vi "S7-PPI协议.vi"() -> ()   [LabVIEW 2014]
uses:
  <vilib>/Instr/_visa.llb/VISA Configure Serial Port (Instr).vi
panel:
  out "RVW34":u16
  out "RVW32":u16
  out "RVW30":u16
  out "RVW28":u16
  out "RVW26":u16
  out "RVW24":u16
  out "RVW22":u16
  out "RVW20":u16
  out "RVW18":u16
  out "RVW16":u16
  out "RVW14":u16
  out "RVW12":u16
  out "RVW10":u16
  out "RVW8":u16
  out "RVW6":u16
  out "RVW4":u16
  out "RVW2":u16
  out "RVW0":u16
  in  "VW34":u16
  in  "VW32":u16
  in  "VW30":u16
  in  "VW28":u16
  in  "VW26":u16
  in  "VW24":u16
  in  "VW22":u16
  in  "VW20":u16
  in  "VW18":u16
  in  "VW16":u16
  in  "VW14":u16
  in  "VW12":u16
  in  "VW10":u16
  in  "VW8":u16
  in  "VW6":u16
  in  "VW4":u16
  in  "VW2":u16
  in  "VW0":u16
  out "值 3":u32
  out "Q3.0":bool
  out "Q3.1":bool
  out "Q3.2":bool
  out "Q3.3":bool
  out "Q3.4":bool
  out "Q3.5":bool
  out "Q3.6":bool
  out "Q3.7":bool
  out "M2.0":bool
  out "M2.1":bool
  out "M2.2":bool
  out "M2.4":bool
  out "M2.3":bool
  out "M2.5":bool
  out "M2.6":bool
  out "M2.7":bool
  out "M1.0":bool
  out "M1.1":bool
  out "M1.2":bool
  out "M1.3":bool
  out "M1.4":bool
  out "M1.5":bool
  out "M1.6":bool
  out "M1.7":bool
  out "M0.0":bool
  out "M0.1":bool
  out "M0.2":bool
  out "M0.3":bool
  out "M0.4":bool
  out "M0.5":bool
  out "M0.6":bool
  out "M0.7":bool
  in  "Q3.0":bool
  in  "Q3.1":bool
  in  "Q3.2":bool
  in  "Q3.3":bool
  in  "Q3.4":bool
  in  "Q3.5":bool
  in  "Q3.6":bool
  in  "Q3.7":bool
  in  "M2.0":bool
  in  "M2.1":bool
  in  "M2.2":bool
  in  "M2.3":bool
  in  "M2.4":bool
  in  "M2.5":bool
  in  "M2.6":bool
  in  "M2.7":bool
  in  "M1.0":bool
  in  "M1.1":bool
  in  "M1.2":bool
  in  "M1.3":bool
  in  "M1.4":bool
  in  "M1.5":bool
  in  "M1.6":bool
  in  "M1.7":bool
  in  "M0.0":bool
  in  "M0.1":bool
  in  "M0.2":bool
  in  "M0.3":bool
  in  "M0.4":bool
  in  "M0.5":bool
  in  "M0.6":bool
  in  "M0.7":bool
  out "值 2":u32
  in  "Q3.0":bool
  in  "Q3.1":bool
  in  "Q3.2":bool
  in  "Q3.3":bool
  in  "Q3.4":bool
  in  "Q3.5":bool
  in  "Q3.6":bool
  in  "Q3.7":bool
  in  "Q2.0":bool
  in  "Q2.1":bool
  in  "Q2.2":bool
  in  "Q2.3":bool
  in  "Q2.4":bool
  in  "Q2.5":bool
  in  "Q2.6":bool
  in  "Q2.7":bool
  in  "Q1.7":bool
  in  "Q1.6":bool
  in  "Q1.5":bool
  in  "Q1.4":bool
  in  "Q1.3":bool
  in  "Q1.2":bool
  in  "Q1.1":bool
  in  "Q1.0":bool
  in  "Q0.7":bool
  in  "Q0.6":bool
  in  "Q0.5":bool
  in  "Q0.4":bool
  in  "Q0.3":bool
  in  "Q0.2":bool
  in  "Q0.1":bool
  in  "Q0.0":bool
  out "Q3.0":bool
  out "Q3.1":bool
  out "Q3.2":bool
  out "Q3.3":bool
  out "Q3.4":bool
  out "Q3.5":bool
  out "Q3.6":bool
  out "Q3.7":bool
  out "Q2.0":bool
  out "Q2.1":bool
  out "Q2.2":bool
  out "Q2.4":bool
  out "Q2.3":bool
  out "Q2.5":bool
  out "Q2.6":bool
  out "Q2.7":bool
  out "Q1.0":bool
  out "Q1.1":bool
  out "Q1.2":bool
  out "Q1.3":bool
  out "Q1.4":bool
  out "Q1.5":bool
  out "Q1.6":bool
  out "Q1.7":bool
  out "Q0.0":bool
  out "Q0.1":bool
  out "Q0.2":bool
  out "Q0.3":bool
  out "Q0.4":bool
  out "Q0.5":bool
  out "Q0.6":bool
  out "Q0.7":bool
  out "I3.0":bool
  out "I3.1":bool
  out "I3.2":bool
  out "I3.3":bool
  out "I3.4":bool
  out "I3.5":bool
  out "I3.6":bool
  out "I3.7":bool
  out "I2.0":bool
  out "I2.1":bool
  out "I2.2":bool
  out "I2.4":bool
  out "I2.3":bool
  out "I2.5":bool
  out "I2.6":bool
  out "I2.7":bool
  out "I1.0":bool
  out "I1.1":bool
  out "I1.2":bool
  out "I1.3":bool
  out "I1.4":bool
  out "I1.5":bool
  out "I1.6":bool
  out "I1.7":bool
  out "I0.0":bool
  out "I0.1":bool
  out "I0.2":bool
  out "I0.3":bool
  out "I0.4":bool
  out "I0.5":bool
  out "I0.6":bool
  out "I0.7":bool
  in  "枚举":T1
  in  "读写时间":u32
  in  "baud":u32=9600 caption="波特率"
  in  "COM":refnum<visa-resource-name> caption="端口"
  in  "停止":bool
  in  "STOP":bool
  in  "RUN":bool
  # "I0.0-I0.7"
  # "I1.0-I1.7"
  # "I2.0-I2.7"
  # "I3.0-I3.7"
  # "https://item.taobao.com/item.htm?id=520867234520"
  # "Q0.0-Q0.7"
  # "Q1.0-Q1.7"
  # "Q2.0-Q2.7"
  # "Q3.0-Q3.7"
  # "本程序密码：635410@ ，已经由楼上的工具破解"
  # "M0.0-M0.7"
  # "M1.0-M1.7"
  # "M2.0-M2.7"
  # "M3.0-M3.7"
  # "运行前请选择正确的通讯端口，和\n波特率。注意读写扫描时间的填写\n此程序PLC默认地址为2，其他不能\n通讯连接。"
  # "注意：1:波特率19.2请将读写时间设置大于80，波特率9600请将读写时间设置大于200，禁止187.5运行,建议19.2kbt/s"
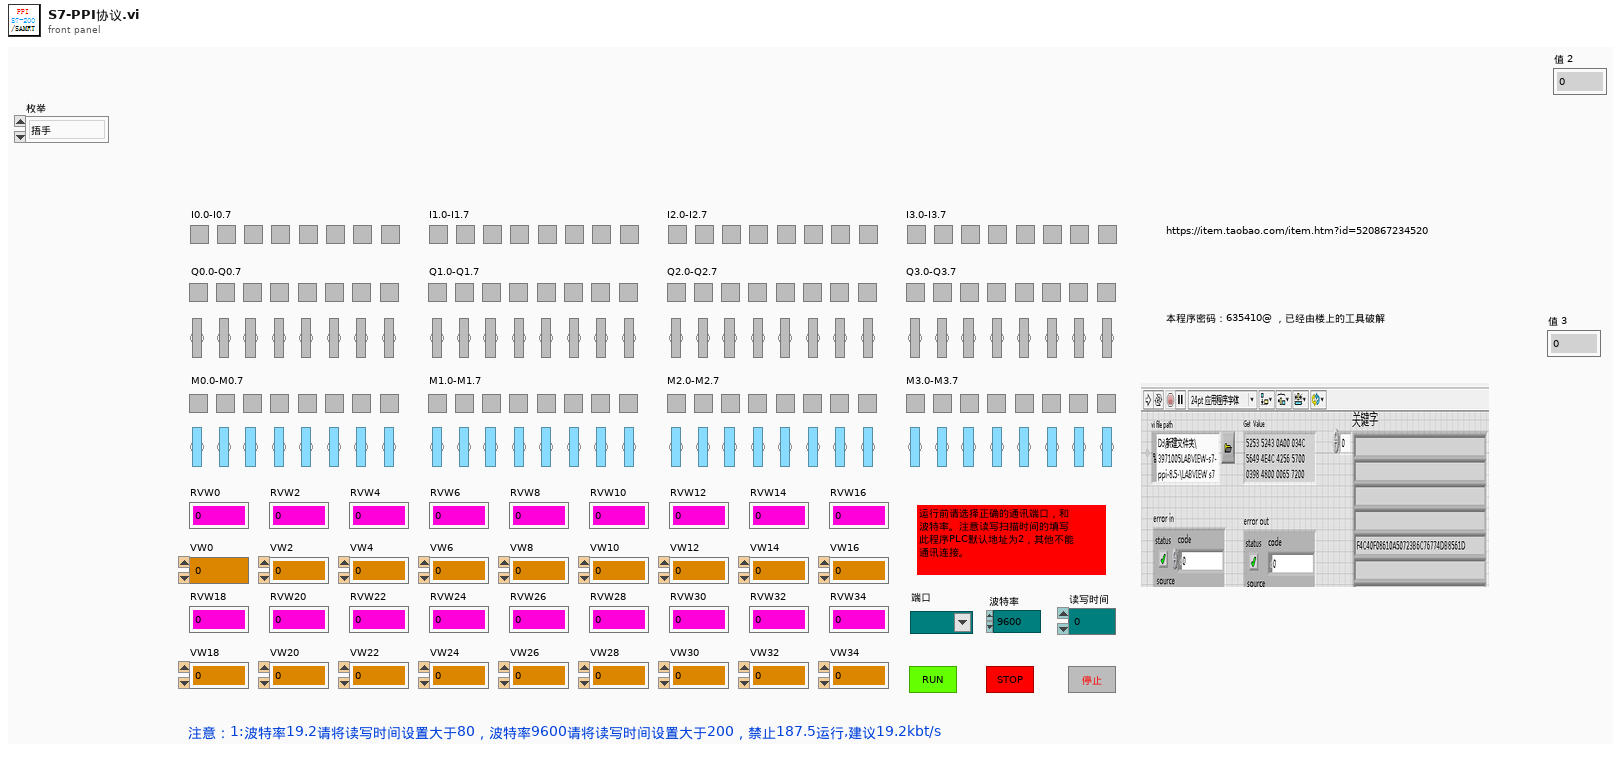
[diagram p1: front panel]
types:
  T1 = typedef "读取值枚举索引.ctl" = enum16{"捂手", "RUN", "STOP", "枚举RI", "枚举RQ", "枚举RM", "枚举RVW", "WID0", "WQD0", "WMD0", "WV"}
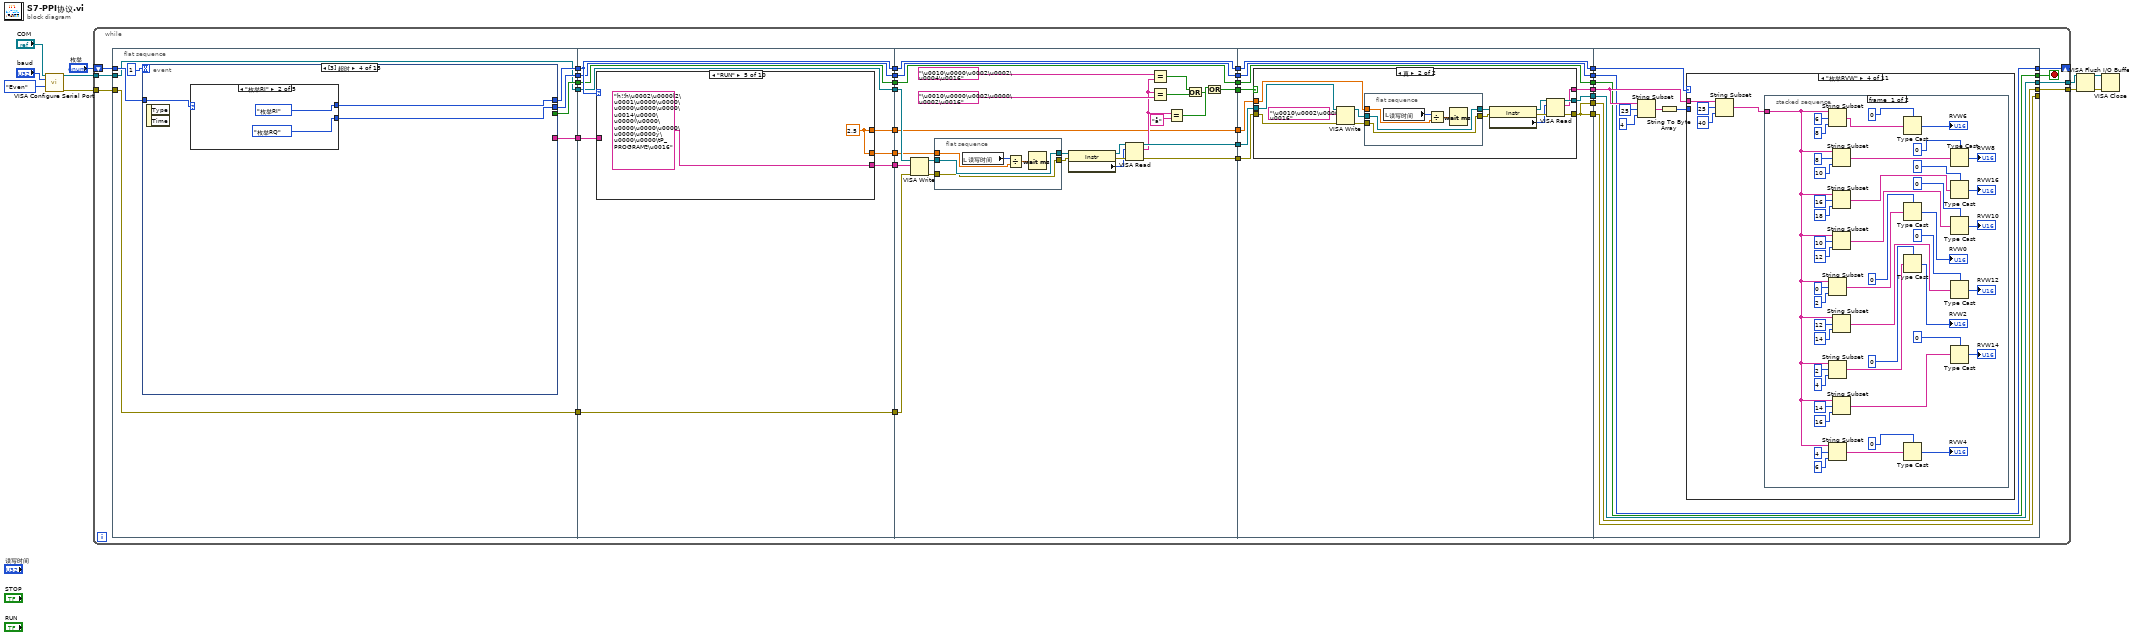
[diagram p0: block diagram]
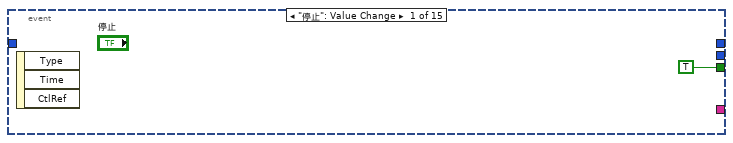
[diagram p2: hidden frame]
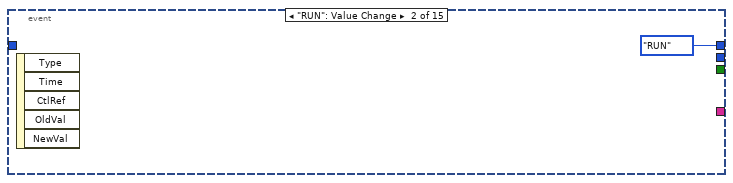
[diagram p3: hidden frame]
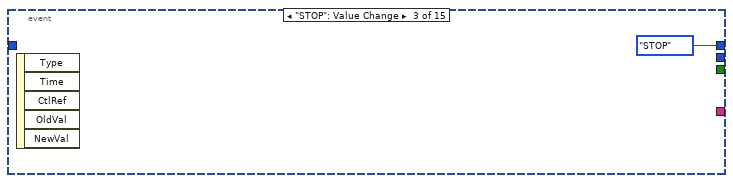
[diagram p4: hidden frame]
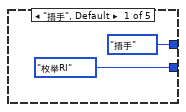
[diagram p5: hidden frame]
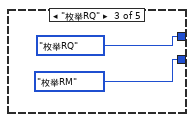
[diagram p6: hidden frame]
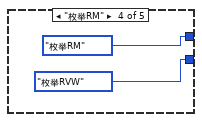
[diagram p7: hidden frame]
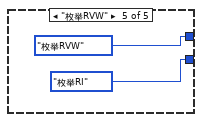
[diagram p8: hidden frame]
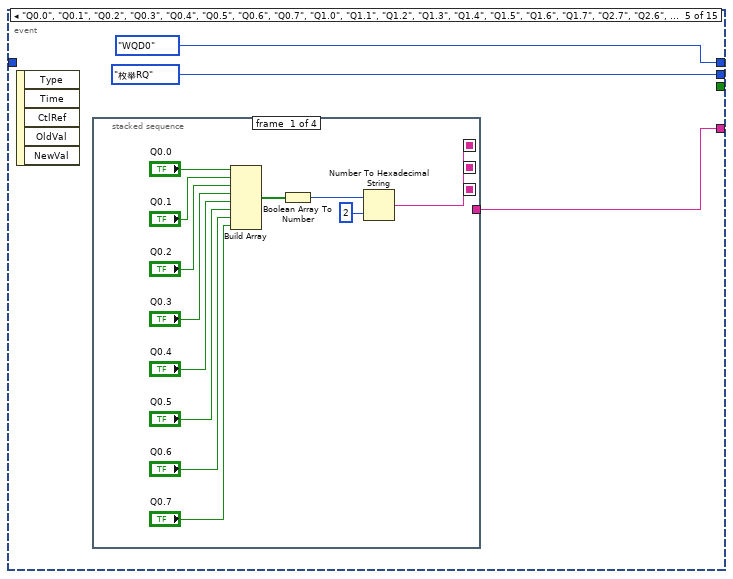
[diagram p9: hidden frame]
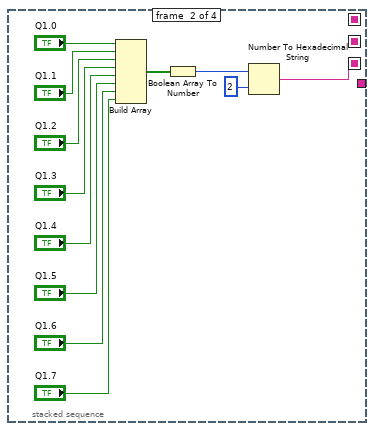
[diagram p10: hidden frame]
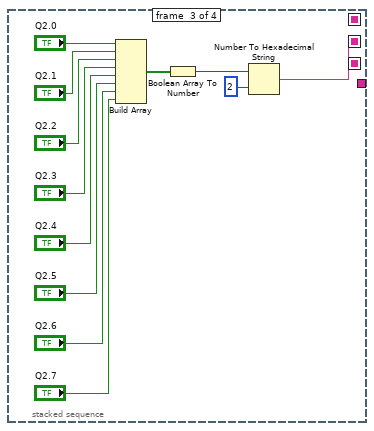
[diagram p11: hidden frame]
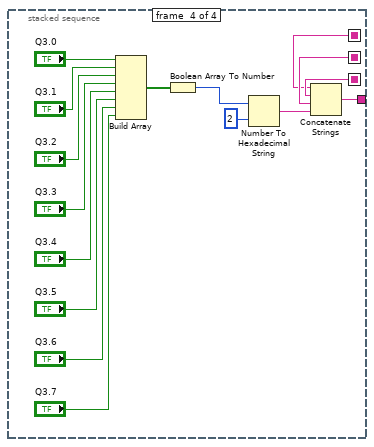
[diagram p12: hidden frame]
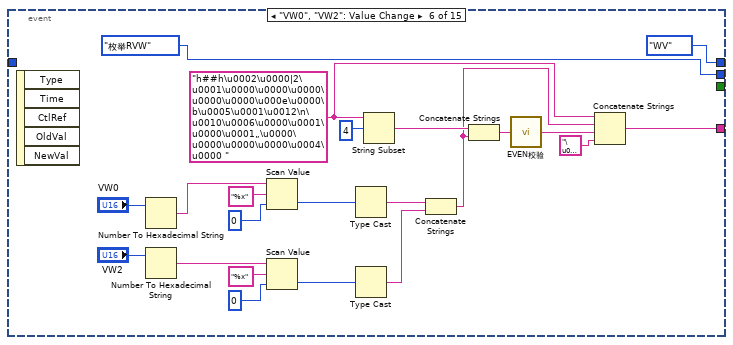
[diagram p13: hidden frame]
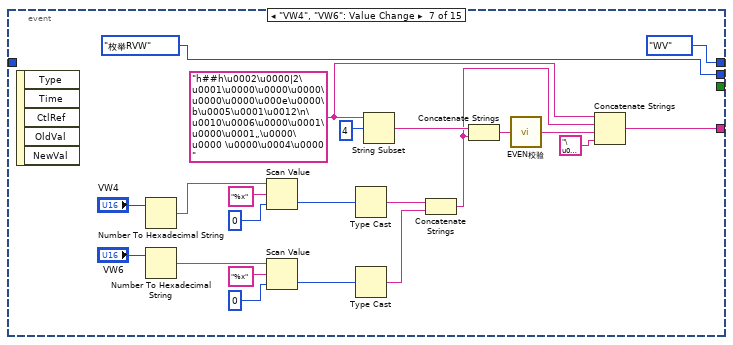
[diagram p14: hidden frame]
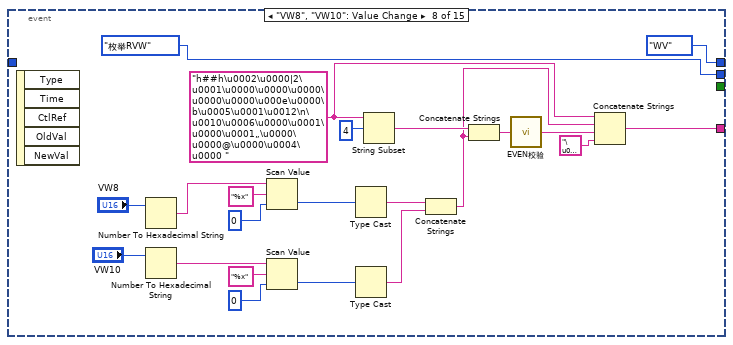
[diagram p15: hidden frame]
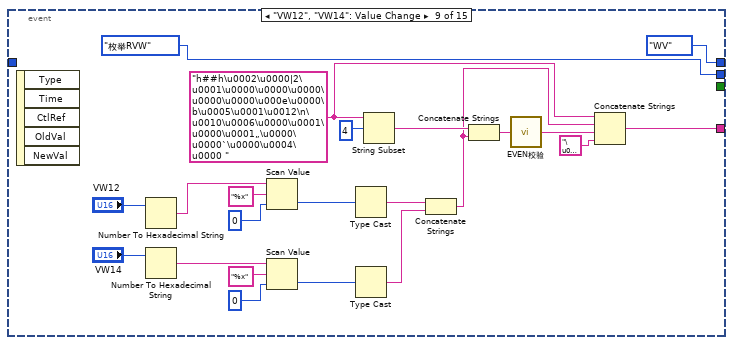
[diagram p16: hidden frame]
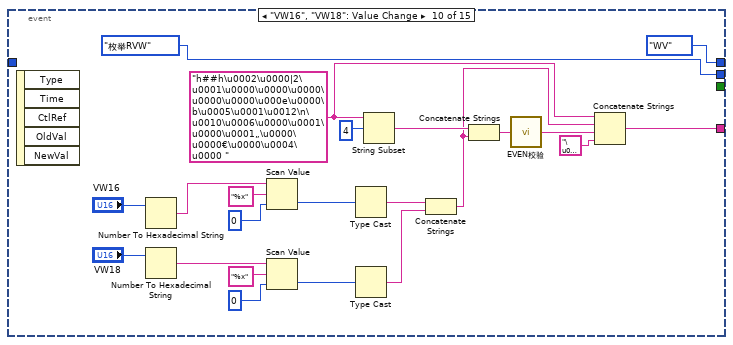
[diagram p17: hidden frame]
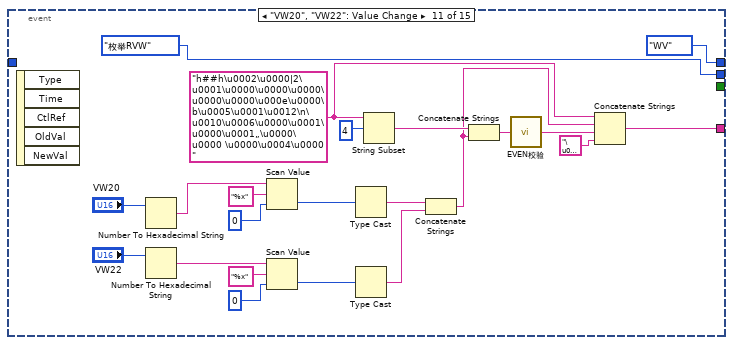
[diagram p18: hidden frame]
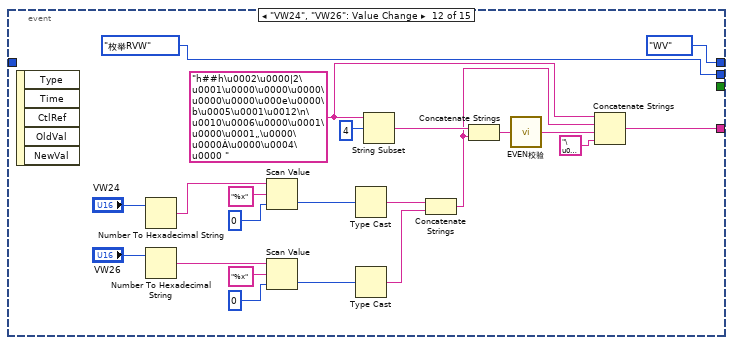
[diagram p19: hidden frame]
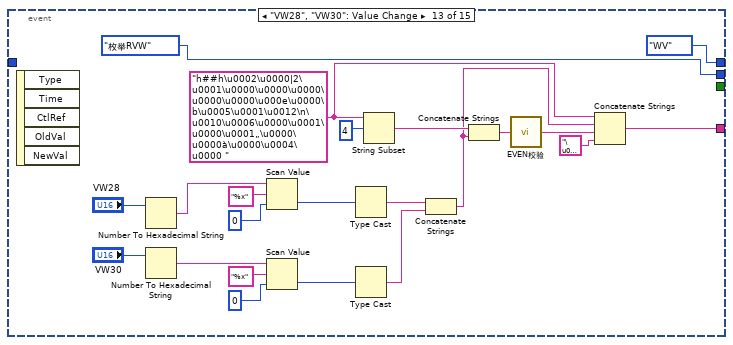
[diagram p20: hidden frame]
diagram:
  n1 = call-poly "VISA Configure Serial Port"("VISA resource name"="COM", "baud rate (9600)"="baud", "parity (0:none)"=enum16{"None", "Odd", "Even", "Mark", "Space"}."Even") -> ("VISA resource name out"=w8:refnum<visa-resource-name>, "error out"=w7:errorcluster)  [unwired: 11 in]
  n2 = while {
    tunnel: w8 -> [w44]
    tunnel: w7 -> [w45]
    shift-right: [w42] -> _
    shift-left: "枚举" -> [w43]
    tunnel: [w40] -> w5
    tunnel: [w39] -> w4
    stop <- w41 stop-if-true
    n3 = flat-sequence {
      tunnel: w45 -> [w47]
      tunnel: w44 -> [w46]
      tunnel: w43 -> [w53]
      tunnel: [w47] -> w38
      tunnel: [w46] -> w37
      tunnel: [w52] -> w36
      tunnel: [w51] -> w35
      tunnel: [w50] -> w34
      tunnel: [w48] -> w33
      tunnel: w38 -> [w381]
      tunnel: w37 -> [w380]
      tunnel: w36 -> [w379]
      tunnel: w35 -> [w385]
      tunnel: w34 -> [w378]
      tunnel: w33 -> [w384]
      tunnel: [w381] -> w32
      tunnel: [w380] -> w31
      tunnel: [w379] -> w30
      tunnel: [w378] -> w29
      tunnel: [w386] -> w28
      tunnel: [w385] -> w27
      tunnel: [w383] -> w26
      tunnel: [w382] -> w25
      tunnel: w32 -> [w446]
      tunnel: w31 -> [w444]
      tunnel: w30 -> [w433]
      tunnel: w29 -> [w432]
      tunnel: w28 -> [w435]
      tunnel: w27 -> [w431]
      tunnel: w26 -> [w434]
      tunnel: w25 -> [w430]
      tunnel: [w433] -> w24
      tunnel: [w455] -> w23
      tunnel: [w454] -> w22
      tunnel: [w441] -> w21
      tunnel: [w432] -> w20
      tunnel: [w431] -> w19
      tunnel: [w430] -> w18
      tunnel: w24 -> [w462]
      tunnel: w23 -> [w469]
      tunnel: w22 -> [w468]
      tunnel: w21 -> [w470]
      tunnel: w20 -> [w463]
      tunnel: w19 -> [w461]
      tunnel: w18 -> [w464]
      tunnel: [w467] -> w17
      tunnel: [w466] -> w16
      tunnel: [w463] -> w15
      tunnel: [w462] -> w14
      tunnel: [w466] -> w13
      tunnel: [w465] -> w12
      tunnel: [w461] -> w11
      tunnel: [w496] -> w40
      tunnel: [w495] -> _
      tunnel: [w494] -> w42
      tunnel: [w493] -> w41
      tunnel: [w492] -> w39
      tunnel: w17 -> [w496]
      tunnel: w16 -> [w495]
      tunnel: w15 -> [w494]
      tunnel: w14 -> [w493]
      tunnel: w13 -> [w492]
      tunnel: w12 -> [w497]
      tunnel: w11 -> [w498]
      frame #0 {
        n4 = event shown="[3] 超时" {
          selector: _ -> [_ _ _ _ _ _ _ _ _ _ _ _ _ _ _]
          dyn-events: _ -> [_ _ _ _ _ _ _ _ _ _ _ _ _ _ _]
          timeout: 1 -> [_ _ _ _ _ _ _ _ _ _ _ _ _ _ _]
          tunnel: w53 -> [_ _ _ w59 _ _ _ _ _ _ _ _ _ _ _]
          tunnel: [_ 读取值枚举索引."RUN" ("枚举 2") 读取值枚举索引."STOP" ("枚举 2") w58 读取值枚举索引."WQD0" ("枚举 2") 读取值枚举索引."WV" ("枚举 2") 读取值枚举索引."WV" ("枚举 2") 读取值枚举索引."WV" ("枚举 2") 读取值枚举索引."WV" ("枚举 2") 读取值枚举索引."WV" ("枚举 2") 读取值枚举索引."WV" ("枚举 2") 读取值枚举索引."WV" ("枚举 2") 读取值枚举索引."WV" ("枚举 2") 读取值枚举索引."WV" ("枚举 2") 读取值枚举索引."WMD0" ("枚举 2")] -> w51
          tunnel: [TRUE _ _ _ _ _ _ _ _ _ _ _ _ _ _] -> w52
          tunnel: [_ _ _ w57 读取值枚举索引."枚举RQ" ("枚举 2") 读取值枚举索引."枚举RVW" ("枚举 2") 读取值枚举索引."枚举RVW" ("枚举 2") 读取值枚举索引."枚举RVW" ("枚举 2") 读取值枚举索引."枚举RVW" ("枚举 2") 读取值枚举索引."枚举RVW" ("枚举 2") 读取值枚举索引."枚举RVW" ("枚举 2") 读取值枚举索引."枚举RVW" ("枚举 2") 读取值枚举索引."枚举RVW" ("枚举 2") 读取值枚举索引."枚举RVW" ("枚举 2") 读取值枚举索引."枚举RM" ("枚举 2")] -> w50
          tunnel: [_ _ _ _ w70 w131 w153 w175 w197 w220 w241 w263 w283 w306 w325] -> w48
          event "停止": Value Change {
            n5 = event-data() -> ()  [unwired: 1 in, 3 out]
          }
          event "RUN": Value Change {
            n6 = event-data() -> ()  [unwired: 1 in, 5 out]
          }
          event "STOP": Value Change {
            n7 = event-data() -> ()  [unwired: 1 in, 5 out]
          }
          event Timeout {
            n8 = event-data() -> ()  [unwired: 1 in, 2 out]
            n9 = case shown="\"枚举RI\"" w59 {
              tunnel: [读取值枚举索引."捂手" ("枚举 2") 读取值枚举索引."枚举RI" ("枚举 2") 读取值枚举索引."枚举RQ" ("枚举 2") 读取值枚举索引."枚举RM" ("枚举 2") 读取值枚举索引."枚举RVW" ("枚举 2")] -> w58
              tunnel: [读取值枚举索引."枚举RI" ("枚举 2") 读取值枚举索引."枚举RQ" ("枚举 2") 读取值枚举索引."枚举RM" ("枚举 2") 读取值枚举索引."枚举RVW" ("枚举 2") 读取值枚举索引."枚举RI" ("枚举 2")] -> w57
              frame "捂手", Default {
              }
              frame "枚举RI" {
              }
              frame "枚举RQ" {
              }
              frame "枚举RM" {
              }
              frame "枚举RVW" {
              }
            }
          }
          event "Q0.0", "Q0.1", "Q0.2", "Q0.3", "Q0.4", "Q0.5", "Q0.6", "Q0.7", "Q1.0", "Q1.1", "Q1.2", "Q1.3", "Q1.4", "Q1.5", "Q1.6", "Q1.7", "Q2.7", "Q2.6", "Q2.5", "Q2.4", "Q2.3", "Q2.2", "Q2.1", "Q2.0", "Q3.7", "Q3.5", "Q3.4", "Q3.3", "Q3.2", "Q3.1", "Q3.0": Value Change {
            n10 = event-data() -> ()  [unwired: 1 in, 5 out]
            n11 = stacked-sequence {
              seq-local: [w73 _ _ _] -> [_ _ _ w110]
              seq-local: [_ w85 _ _] -> [_ _ _ w113]
              seq-local: [_ _ w97 _] -> [_ _ _ w112]
              tunnel: [_ _ _ w109] -> w70
              frame #0 {
                n12 = Build Array("Q0.0", "Q0.1", "Q0.2", "Q0.3", "Q0.4", "Q0.5", "Q0.6", "Q0.7") -> (w84:bool[])
                n13 = Boolean Array To Number(Boolean array=w84) -> (number=w82:u32)
                n14 = Number To Hexadecimal String(1:i16 2 ("宽度(-)"), 2:w82) -> (0:w73:string)
              }
              frame #1 {
                n15 = Build Array("Q1.0", "Q1.1", "Q1.2", "Q1.3", "Q1.4", "Q1.5", "Q1.6", "Q1.7") -> (w96:bool[])
                n16 = Boolean Array To Number(Boolean array=w96) -> (number=w94:u32)
                n17 = Number To Hexadecimal String(1:i16 2 ("宽度(-)"), 2:w94) -> (0:w85:string)
              }
              frame #2 {
                n18 = Build Array("Q2.0", "Q2.1", "Q2.2", "Q2.3", "Q2.4", "Q2.5", "Q2.6", "Q2.7") -> (w108:bool[])
                n19 = Boolean Array To Number(Boolean array=w108) -> (number=w106:u32)
                n20 = Number To Hexadecimal String(1:i16 2 ("宽度(-)"), 2:w106) -> (0:w97:string)
              }
              frame #3 {
                n21 = Build Array("Q3.0", "Q3.1", "Q3.2", "Q3.3", "Q3.4", "Q3.5", "Q3.6", "Q3.7") -> (w122:bool[])
                n22 = Boolean Array To Number(Boolean array=w122) -> (number=w124:u32)
                n23 = Number To Hexadecimal String(1:i16 2 ("宽度(-)"), 2:w124) -> (0:w111:string)
                n24 = Concatenate Strings(w110, w113, w112, w111) -> (w109:string)
              }
            }
          }
          event "VW0", "VW2": Value Change {
            w126 = "h##h\u0002\u0000|2\u0001\u0000\u0000\u0000\u0000\u0000\u000e\u0000\b\u0005\u0001\u0012\n\u0010\u0006\u0000\u0001\u0000\u0001„\u0000\u0000\u0000\u0000\u0004\u0000 "
            n25 = event-data() -> ()  [unwired: 1 in, 5 out]
            n26 = Number To Hexadecimal String(2:"VW0") -> (0:w141:string)  [unwired: 1 in]
            n27 = Number To Hexadecimal String(2:"VW2") -> (0:w146:string)  [unwired: 1 in]
            n28 = Scan Value(string=w141, format string="%x" ("格式字符串"), default (0 dbl)=u16 0 ("默认(0 dbl)")) -> (value=w142:u16)  [unwired: 1 out]
            n29 = Scan Value(string=w146, format string="%x" ("格式字符串"), default (0 dbl)=u16 0 ("默认(0 dbl)")) -> (value=w143:u16)  [unwired: 1 out]
            n30 = Type Cast(x=w142) -> (*(type *) &x=w128:string)  [unwired: 1 in]
            n31 = Type Cast(x=w143) -> (*(type *) &x=w127:string)  [unwired: 1 in]
            n32 = String Subset(string=w126, offset (0)=4 ("偏移量(0)")) -> (substring=w135:string)  [unwired: 1 in]
            n33 = Concatenate Strings(w128, w127) -> (w125:string)
            n34 = Concatenate Strings(w135, w125) -> (w132:string)
            n35 = call "EVEN校验.vi"("校验字符串"=w132) -> ("校验码"=w134:string)
            n36 = Concatenate Strings(w126, w125, w134, "\u0016" ("字符串")) -> (w131:string)
          }
          event "VW4", "VW6": Value Change {
            w150 = "h##h\u0002\u0000|2\u0001\u0000\u0000\u0000\u0000\u0000\u000e\u0000\b\u0005\u0001\u0012\n\u0010\u0006\u0000\u0001\u0000\u0001„\u0000\u0000 \u0000\u0004\u0000 "
            n37 = event-data() -> ()  [unwired: 1 in, 5 out]
            n38 = Number To Hexadecimal String(2:"VW4") -> (0:w168:string)  [unwired: 1 in]
            n39 = Number To Hexadecimal String(2:"VW6") -> (0:w163:string)  [unwired: 1 in]
            n40 = Scan Value(string=w168, format string="%x" ("格式字符串"), default (0 dbl)=u16 0 ("默认(0 dbl)")) -> (value=w165:u16)  [unwired: 1 out]
            n41 = Scan Value(string=w163, format string="%x" ("格式字符串"), default (0 dbl)=u16 0 ("默认(0 dbl)")) -> (value=w164:u16)  [unwired: 1 out]
            n42 = Type Cast(x=w165) -> (*(type *) &x=w147:string)  [unwired: 1 in]
            n43 = Type Cast(x=w164) -> (*(type *) &x=w148:string)  [unwired: 1 in]
            n44 = String Subset(string=w150, offset (0)=4 ("偏移量(0)")) -> (substring=w159:string)  [unwired: 1 in]
            n45 = Concatenate Strings(w147, w148) -> (w149:string)
            n46 = Concatenate Strings(w159, w149) -> (w156:string)
            n47 = call "EVEN校验.vi"("校验字符串"=w156) -> ("校验码"=w158:string)
            n48 = Concatenate Strings(w150, w149, w158, "\u0016" ("字符串")) -> (w153:string)
          }
          event "VW8", "VW10": Value Change {
            w172 = "h##h\u0002\u0000|2\u0001\u0000\u0000\u0000\u0000\u0000\u000e\u0000\b\u0005\u0001\u0012\n\u0010\u0006\u0000\u0001\u0000\u0001„\u0000\u0000@\u0000\u0004\u0000 "
            n49 = event-data() -> ()  [unwired: 1 in, 5 out]
            n50 = Number To Hexadecimal String(2:"VW8") -> (0:w190:string)  [unwired: 1 in]
            n51 = Number To Hexadecimal String(2:"VW10") -> (0:w185:string)  [unwired: 1 in]
            n52 = Scan Value(string=w190, format string="%x" ("格式字符串"), default (0 dbl)=u16 0 ("默认(0 dbl)")) -> (value=w187:u16)  [unwired: 1 out]
            n53 = Scan Value(string=w185, format string="%x" ("格式字符串"), default (0 dbl)=u16 0 ("默认(0 dbl)")) -> (value=w186:u16)  [unwired: 1 out]
            n54 = Type Cast(x=w187) -> (*(type *) &x=w169:string)  [unwired: 1 in]
            n55 = Type Cast(x=w186) -> (*(type *) &x=w170:string)  [unwired: 1 in]
            n56 = String Subset(string=w172, offset (0)=4 ("偏移量(0)")) -> (substring=w181:string)  [unwired: 1 in]
            n57 = Concatenate Strings(w169, w170) -> (w171:string)
            n58 = Concatenate Strings(w181, w171) -> (w178:string)
            n59 = call "EVEN校验.vi"("校验字符串"=w178) -> ("校验码"=w180:string)
            n60 = Concatenate Strings(w172, w171, w180, "\u0016" ("字符串")) -> (w175:string)
          }
          event "VW12", "VW14": Value Change {
            w194 = "h##h\u0002\u0000|2\u0001\u0000\u0000\u0000\u0000\u0000\u000e\u0000\b\u0005\u0001\u0012\n\u0010\u0006\u0000\u0001\u0000\u0001„\u0000\u0000`\u0000\u0004\u0000 "
            n61 = event-data() -> ()  [unwired: 1 in, 5 out]
            n62 = Number To Hexadecimal String(2:"VW12") -> (0:w212:string)  [unwired: 1 in]
            n63 = Number To Hexadecimal String(2:"VW14") -> (0:w207:string)  [unwired: 1 in]
            n64 = Scan Value(string=w212, format string="%x" ("格式字符串"), default (0 dbl)=u16 0 ("默认(0 dbl)")) -> (value=w209:u16)  [unwired: 1 out]
            n65 = Scan Value(string=w207, format string="%x" ("格式字符串"), default (0 dbl)=u16 0 ("默认(0 dbl)")) -> (value=w208:u16)  [unwired: 1 out]
            n66 = Type Cast(x=w209) -> (*(type *) &x=w192:string)  [unwired: 1 in]
            n67 = Type Cast(x=w208) -> (*(type *) &x=w191:string)  [unwired: 1 in]
            n68 = String Subset(string=w194, offset (0)=4 ("偏移量(0)")) -> (substring=w203:string)  [unwired: 1 in]
            n69 = Concatenate Strings(w192, w191) -> (w193:string)
            n70 = Concatenate Strings(w203, w193) -> (w200:string)
            n71 = call "EVEN校验.vi"("校验字符串"=w200) -> ("校验码"=w202:string)
            n72 = Concatenate Strings(w194, w193, w202, "\u0016" ("字符串")) -> (w197:string)
          }
          event "VW16", "VW18": Value Change {
            w215 = "h##h\u0002\u0000|2\u0001\u0000\u0000\u0000\u0000\u0000\u000e\u0000\b\u0005\u0001\u0012\n\u0010\u0006\u0000\u0001\u0000\u0001„\u0000\u0000€\u0000\u0004\u0000 "
            n73 = event-data() -> ()  [unwired: 1 in, 5 out]
            n74 = Number To Hexadecimal String(2:"VW16") -> (0:w229:string)  [unwired: 1 in]
            n75 = Number To Hexadecimal String(2:"VW18") -> (0:w234:string)  [unwired: 1 in]
            n76 = Scan Value(string=w229, format string="%x" ("格式字符串"), default (0 dbl)=u16 0 ("默认(0 dbl)")) -> (value=w230:u16)  [unwired: 1 out]
            n77 = Scan Value(string=w234, format string="%x" ("格式字符串"), default (0 dbl)=u16 0 ("默认(0 dbl)")) -> (value=w231:u16)  [unwired: 1 out]
            n78 = Type Cast(x=w230) -> (*(type *) &x=w217:string)  [unwired: 1 in]
            n79 = Type Cast(x=w231) -> (*(type *) &x=w216:string)  [unwired: 1 in]
            n80 = String Subset(string=w215, offset (0)=4 ("偏移量(0)")) -> (substring=w225:string)  [unwired: 1 in]
            n81 = Concatenate Strings(w217, w216) -> (w213:string)
            n82 = Concatenate Strings(w225, w213) -> (w214:string)
            n83 = call "EVEN校验.vi"("校验字符串"=w214) -> ("校验码"=w224:string)
            n84 = Concatenate Strings(w215, w213, w224, "\u0016" ("字符串")) -> (w220:string)
          }
          event "VW20", "VW22": Value Change {
            w238 = "h##h\u0002\u0000|2\u0001\u0000\u0000\u0000\u0000\u0000\u000e\u0000\b\u0005\u0001\u0012\n\u0010\u0006\u0000\u0001\u0000\u0001„\u0000\u0000 \u0000\u0004\u0000 "
            n85 = event-data() -> ()  [unwired: 1 in, 5 out]
            n86 = Number To Hexadecimal String(2:"VW20") -> (0:w256:string)  [unwired: 1 in]
            n87 = Number To Hexadecimal String(2:"VW22") -> (0:w251:string)  [unwired: 1 in]
            n88 = Scan Value(string=w256, format string="%x" ("格式字符串"), default (0 dbl)=u16 0 ("默认(0 dbl)")) -> (value=w253:u16)  [unwired: 1 out]
            n89 = Scan Value(string=w251, format string="%x" ("格式字符串"), default (0 dbl)=u16 0 ("默认(0 dbl)")) -> (value=w252:u16)  [unwired: 1 out]
            n90 = Type Cast(x=w253) -> (*(type *) &x=w235:string)  [unwired: 1 in]
            n91 = Type Cast(x=w252) -> (*(type *) &x=w236:string)  [unwired: 1 in]
            n92 = String Subset(string=w238, offset (0)=4 ("偏移量(0)")) -> (substring=w247:string)  [unwired: 1 in]
            n93 = Concatenate Strings(w235, w236) -> (w237:string)
            n94 = Concatenate Strings(w247, w237) -> (w244:string)
            n95 = call "EVEN校验.vi"("校验字符串"=w244) -> ("校验码"=w246:string)
            n96 = Concatenate Strings(w238, w237, w246, "\u0016" ("字符串")) -> (w241:string)
          }
          event "VW24", "VW26": Value Change {
            w258 = "h##h\u0002\u0000|2\u0001\u0000\u0000\u0000\u0000\u0000\u000e\u0000\b\u0005\u0001\u0012\n\u0010\u0006\u0000\u0001\u0000\u0001„\u0000\u0000À\u0000\u0004\u0000 "
            n97 = event-data() -> ()  [unwired: 1 in, 5 out]
            n98 = Number To Hexadecimal String(2:"VW24") -> (0:w273:string)  [unwired: 1 in]
            n99 = Number To Hexadecimal String(2:"VW26") -> (0:w278:string)  [unwired: 1 in]
            n100 = Scan Value(string=w273, format string="%x" ("格式字符串"), default (0 dbl)=u16 0 ("默认(0 dbl)")) -> (value=w274:u16)  [unwired: 1 out]
            n101 = Scan Value(string=w278, format string="%x" ("格式字符串"), default (0 dbl)=u16 0 ("默认(0 dbl)")) -> (value=w275:u16)  [unwired: 1 out]
            n102 = Type Cast(x=w274) -> (*(type *) &x=w260:string)  [unwired: 1 in]
            n103 = Type Cast(x=w275) -> (*(type *) &x=w259:string)  [unwired: 1 in]
            n104 = String Subset(string=w258, offset (0)=4 ("偏移量(0)")) -> (substring=w269:string)  [unwired: 1 in]
            n105 = Concatenate Strings(w260, w259) -> (w257:string)
            n106 = Concatenate Strings(w269, w257) -> (w266:string)
            n107 = call "EVEN校验.vi"("校验字符串"=w266) -> ("校验码"=w268:string)
            n108 = Concatenate Strings(w258, w257, w268, "\u0016" ("字符串")) -> (w263:string)
          }
          event "VW28", "VW30": Value Change {
            w280 = "h##h\u0002\u0000|2\u0001\u0000\u0000\u0000\u0000\u0000\u000e\u0000\b\u0005\u0001\u0012\n\u0010\u0006\u0000\u0001\u0000\u0001„\u0000\u0000à\u0000\u0004\u0000 "
            n109 = event-data() -> ()  [unwired: 1 in, 5 out]
            n110 = Number To Hexadecimal String(2:"VW28") -> (0:w293:string)  [unwired: 1 in]
            n111 = Number To Hexadecimal String(2:"VW30") -> (0:w288:string)  [unwired: 1 in]
            n112 = Scan Value(string=w293, format string="%x" ("格式字符串"), default (0 dbl)=u16 0 ("默认(0 dbl)")) -> (value=w292:u16)  [unwired: 1 out]
            n113 = Scan Value(string=w288, format string="%x" ("格式字符串"), default (0 dbl)=u16 0 ("默认(0 dbl)")) -> (value=w291:u16)  [unwired: 1 out]
            n114 = Type Cast(x=w292) -> (*(type *) &x=w282:string)  [unwired: 1 in]
            n115 = Type Cast(x=w291) -> (*(type *) &x=w281:string)  [unwired: 1 in]
            n116 = String Subset(string=w280, offset (0)=4 ("偏移量(0)")) -> (substring=w297:string)  [unwired: 1 in]
            n117 = Concatenate Strings(w282, w281) -> (w279:string)
            n118 = Concatenate Strings(w297, w279) -> (w300:string)
            n119 = call "EVEN校验.vi"("校验字符串"=w300) -> ("校验码"=w298:string)
            n120 = Concatenate Strings(w280, w279, w298, "\u0016" ("字符串")) -> (w283:string)
          }
          event "VW32", "VW34": Value Change {
            w302 = "h##h\u0002\u0000|2\u0001\u0000\u0000\u0000\u0000\u0000\u000e\u0000\b\u0005\u0001\u0012\n\u0010\u0006\u0000\u0001\u0000\u0001„\u0000\u0001\u0000\u0000\u0004\u0000 "
            n121 = event-data() -> ()  [unwired: 1 in, 5 out]
            n122 = Number To Hexadecimal String(2:"VW32") -> (0:w317:string)  [unwired: 1 in]
            n123 = Number To Hexadecimal String(2:"VW34") -> (0:w322:string)  [unwired: 1 in]
            n124 = Scan Value(string=w317, format string="%x" ("格式字符串"), default (0 dbl)=u16 0 ("默认(0 dbl)")) -> (value=w318:u16)  [unwired: 1 out]
            n125 = Scan Value(string=w322, format string="%x" ("格式字符串"), default (0 dbl)=u16 0 ("默认(0 dbl)")) -> (value=w319:u16)  [unwired: 1 out]
            n126 = Type Cast(x=w318) -> (*(type *) &x=w305:string)  [unwired: 1 in]
            n127 = Type Cast(x=w319) -> (*(type *) &x=w304:string)  [unwired: 1 in]
            n128 = String Subset(string=w302, offset (0)=4 ("偏移量(0)")) -> (substring=w314:string)  [unwired: 1 in]
            n129 = Concatenate Strings(w305, w304) -> (w301:string)
            n130 = Concatenate Strings(w314, w301) -> (w311:string)
            n131 = call "EVEN校验.vi"("校验字符串"=w311) -> ("校验码"=w313:string)
            n132 = Concatenate Strings(w302, w301, w313, "\u0016" ("字符串")) -> (w306:string)
          }
          event "M1.7", "M0.6", "M0.5", "M0.4", "M0.3", "M0.2", "M0.1", "M0.0", "M1.6", "M1.5", "M1.4", "M1.3", "M1.2", "M1.1", "M0.7", "M1.0", "M2.7", "M2.6", "M2.5", "M2.4", "M2.3", "M2.2", "M2.1", "M2.0", "Q3.7", "Q3.6", "Q3.5", "Q3.4", "Q3.3", "Q3.2", "Q3.1", "Q3.0": Value Change {
            n133 = event-data() -> ()  [unwired: 1 in, 5 out]
            n134 = stacked-sequence {
              seq-local: [w326 _ _ _] -> [_ _ _ w363]
              seq-local: [_ w338 _ _] -> [_ _ _ w366]
              seq-local: [_ _ w350 _] -> [_ _ _ w365]
              tunnel: [_ _ _ w362] -> w325
              frame #0 {
                n135 = Build Array("M0.0", "M0.1", "M0.2", "M0.3", "M0.4", "M0.5", "M0.6", "M0.7") -> (w337:bool[])
                n136 = Boolean Array To Number(Boolean array=w337) -> (number=w335:u32)
                n137 = Number To Hexadecimal String(1:i16 2 ("宽度(-)"), 2:w335) -> (0:w326:string)
              }
              frame #1 {
                n138 = Build Array("M1.0", "M1.1", "M1.2", "M1.3", "M1.4", "M1.5", "M1.6", "M1.7") -> (w349:bool[])
                n139 = Boolean Array To Number(Boolean array=w349) -> (number=w347:u32)
                n140 = Number To Hexadecimal String(1:i16 2 ("宽度(-)"), 2:w347) -> (0:w338:string)
              }
              frame #2 {
                n141 = Build Array("M2.0", "M2.1", "M2.2", "M2.3", "M2.4", "M2.5", "M2.6", "M2.7") -> (w361:bool[])
                n142 = Boolean Array To Number(Boolean array=w361) -> (number=w359:u32)
                n143 = Number To Hexadecimal String(1:i16 2 ("宽度(-)"), 2:w359) -> (0:w350:string)
              }
              frame #3 {
                n144 = Build Array("Q3.0", "Q3.1", "Q3.2", "Q3.3", "Q3.4", "Q3.5", "Q3.6", "Q3.7") -> (w375:bool[])
                n145 = Boolean Array To Number(Boolean array=w375) -> (number=w377:u32)
                n146 = Number To Hexadecimal String(1:i16 2 ("宽度(-)"), 2:w377) -> (0:w364:string)
                n147 = Concatenate Strings(w363, w366, w365, w364) -> (w362:string)
              }
            }
          }
        }
      }
      frame #1 {
        n148 = case shown="\"RUN\"" w385 {
          tunnel: ["\u0010\u0002\u0000IK\u0016" ("写入缓冲区") "h\u001b\u001bh\u0002\u0000l2\u0001\u0000\u0000\u0000\u0000\u0000\u000e\u0000\u0000\u0004\u0001\u0012\n\u0010\u0006\u0000\u0001\u0000\u0000\u0000\u0000\u0000h\u0016" ("写入缓冲区") "h\u001b\u001bh\u0002\u0000l2\u0001\u0000\u0000\u0000\u0000\u0000\u000e\u0000\u0000\u0004\u0001\u0012\n\u0010\u0006\u0000\u0001\u0000\u0000‚\u0000\u0000\u0000i\u0016" ("写入缓冲区") "h\u001b\u001bh\u0002\u0000l2\u0001\u0000\u0000\u0000\u0000\u0000\u000e\u0000\u0000\u0004\u0001\u0012\n\u0010\u0006\u0000\u0001\u0000\u0000ƒ\u0000\u0000\u0000j\u0016" ("写入缓冲区") "h!!h\u0002\u0000l2\u0001\u0000\u0000\u0000\u0000\u0000\u0014\u0000\u0000(\u0000\u0000\u0000\u0000\u0000\u0000ý\u0000\u0000\tP_PROGRAMª\u0016" "h\u001d\u001dh\u0002\u0000l2\u0001\u0000\u0000\u0000\u0000\u0000\u0010\u0000\u0000)\u0000\u0000\u0000\u0000\u0000\tP_PROGRAMª\u0016" w405 w413 w426 "h\u001b\u001bh\u0002\u0000l2\u0001\u0000\u0000\u0000\u0000\u0000\u000e\u0000\u0000\u0004\u0001\u0012\n\u0010\u0006\u0000\n\u0000\u0001„\u0000\u0000\u0000u\u0016" ("写入缓冲区")] -> w386
          tunnel: w384 -> [_ _ _ _ _ _ w401 w414 w426 _]
          tunnel: [w387 w389 w391 w393 w395 w397 w399 w412 w425 2.0 ("y")] -> w383
          tunnel: [w387 w389 w391 w393 w395 w397 w399 w412 w425 1.0 ("y")] -> w382
          frame "捂手", Default {
            w387 = 2.5 ("y")
          }
          frame "枚举RI" {
            w389 = 2.5 ("y")
          }
          frame "枚举RQ" {
            w391 = 2.5 ("y")
          }
          frame "枚举RM" {
            w393 = 2.5 ("y")
          }
          frame "RUN" {
            w395 = 2.5 ("y")
          }
          frame "STOP" {
            w397 = 2.5 ("y")
          }
          frame "WQD0" {
            w399 = 2.5 ("y")
            w408 = "h##h\u0002\u0000|2\u0001\u0000\u0000\u0000\u0000\u0000\u000e\u0000\b\u0005\u0001\u0012\n\u0010\u0006\u0000\u0001\u0000\u0000‚\u0000\u0000\u0000\u0000\u0004\u0000 "
            n149 = Scan Value(string=w401, format string="%x" ("格式字符串"), default (0 dbl)=u32 0 ("默认(0 dbl)")) -> (value=w404:u32)  [unwired: 1 out]
            "值 2" <- w404
            n150 = Type Cast(x=w404) -> (*(type *) &x=w400:string)  [unwired: 1 in]
            n151 = String Subset(string=w408, offset (0)=4 ("偏移量(0)")) -> (substring=w410:string)  [unwired: 1 in]
            n152 = Concatenate Strings(w410, w400) -> (w409:string)
            n153 = call "EVEN校验.vi"("校验字符串"=w409) -> ("校验码"=w407:string)
            n154 = Concatenate Strings(w408, w400, w407, "\u0016" ("字符串")) -> (w405:string)
          }
          frame "WMD0" {
            w412 = 2.5 ("y")
            w421 = "h##h\u0002\u0000|2\u0001\u0000\u0000\u0000\u0000\u0000\u000e\u0000\b\u0005\u0001\u0012\n\u0010\u0006\u0000\u0001\u0000\u0000ƒ\u0000\u0000\u0000\u0000\u0004\u0000 "
            n155 = Scan Value(string=w414, format string="%x" ("格式字符串"), default (0 dbl)=u32 0 ("默认(0 dbl)")) -> (value=w418:u32)  [unwired: 1 out]
            "值 3" <- w418
            n156 = Type Cast(x=w418) -> (*(type *) &x=w415:string)  [unwired: 1 in]
            n157 = String Subset(string=w421, offset (0)=4 ("偏移量(0)")) -> (substring=w423:string)  [unwired: 1 in]
            n158 = Concatenate Strings(w423, w415) -> (w422:string)
            n159 = call "EVEN校验.vi"("校验字符串"=w422) -> ("校验码"=w420:string)
            n160 = Concatenate Strings(w421, w415, w420, "\u0016" ("字符串")) -> (w413:string)
          }
          frame "WV" {
            w425 = 2.5 ("y")
          }
          frame "枚举RVW" {
          }
        }
      }
      frame #2 {
        n161 = VISA Write(VISA resource name=w444, write buffer=w435, error in (no error)=w446) -> (VISA resource name out=w450:refnum<visa-resource-name>, error out=w447:errorcluster)  [unwired: 1 out]
        n162 = flat-sequence {
          tunnel: w450 -> [w458]
          tunnel: [w458] -> w449
          tunnel: [w457] -> w448
          tunnel: w447 -> [w457]
          tunnel: w434 -> [w456]
          frame #0 {
            n163 = local read "读写时间"() -> (w459:u32)
            n164 = Divide(x=w459, y=w456) -> (x/y=w460:dbl)
            n165 = Wait (ms)(milliseconds to wait=w460) -> ()  [unwired: 1 out]
          }
        }
        n166 = property class="Instr"(reference=w449, error in=w448) -> (reference out=w451:refnum<visa-resource-name>, error out=w453:errorcluster, "Serial Settings:Number of Bytes at Serial Port"=w452:u32)
        n167 = VISA Read(VISA resource name=w451, byte count=w452, error in (no error)=w453) -> (VISA resource name out=w455:refnum<visa-resource-name>, read buffer=w440:string, error out=w454:errorcluster)  [unwired: 1 out]
        n168 = Equal?(x="\u0010\u0000\u0002\u0002\u0004\u0016" ("y"), y=w440) -> (x = y?=w438:bool)
        n169 = Equal?(x=w440, y="\u0010\u0000\u0002\u0000\u0002\u0016") -> (x = y?=w437:bool)
        n170 = Equal?(x=w440, y="å") -> (x = y?=w442:bool)
        n171 = Or(x=w438, y=w437) -> (x .or. y?=w436:bool)
        n172 = Or(x=w442, y=w436) -> (x .or. y?=w441:bool)
      }
      frame #3 {
        n173 = case shown="真" w470 {
          tunnel: [w472 w486] -> w467
          tunnel: [w471 w475] -> w466
          tunnel: w469 -> [w472 w477]
          tunnel: w468 -> [w471 w476]
          tunnel: [_ w474] -> w465
          tunnel: w464 -> [_ w473]
          frame False {
          }
          frame True {
            n174 = VISA Write(VISA resource name=w477, write buffer="\u0010\u0002\u0000\\^\u0016" ("写入缓冲区"), error in (no error)=w476) -> (VISA resource name out=w482:refnum<visa-resource-name>, error out=w479:errorcluster)  [unwired: 1 out]
            n175 = flat-sequence {
              tunnel: w482 -> [w489]
              tunnel: [w489] -> w481
              tunnel: [w488] -> w480
              tunnel: w479 -> [w488]
              tunnel: w473 -> [w487]
              frame #0 {
                n176 = local read "读写时间"() -> (w490:u32)
                n177 = Divide(x=w490, y=w487) -> (x/y=w491:dbl)
                n178 = Wait (ms)(milliseconds to wait=w491) -> ()  [unwired: 1 out]
              }
            }
            n179 = property class="Instr"(reference=w481, error in=w480) -> (reference out=w483:refnum<visa-resource-name>, error out=w485:errorcluster, "Serial Settings:Number of Bytes at Serial Port"=w484:u32)
            n180 = VISA Read(VISA resource name=w483, byte count=w484, error in (no error)=w485) -> (VISA resource name out=w486:refnum<visa-resource-name>, read buffer=w474:string, error out=w475:errorcluster)  [unwired: 1 out]
          }
        }
      }
      frame #4 {
        n181 = String Subset(string=w497, offset (0)=25 ("偏移量(0)"), length (rest)=4 ("长度（剩余）")) -> (substring=w500:string)
        n182 = String To Byte Array(string=w500) -> (unsigned byte array=w499:u8[])
        n183 = case shown="\"枚举RVW\"" w498 {
          tunnel: w499 -> [w503 w584 w665 _ _ _ _ _ _ _ _]
          tunnel: w497 -> [_ _ _ w747 _ _ _ _ _ _ _]
          frame "枚举RI" {
            n184 = stacked-sequence {
              seq-local: [w508 _ _ _] -> [_ w533 _ _]
              seq-local: [w506 _ _ _] -> [_ _ w550 _]
              seq-local: [w504 _ _ _] -> [_ _ _ w567]
              tunnel: w503 -> [w515 _ _ _]
              frame #0 {
                n185 = Index Array(array=w515, index=1 ("索引")) -> (element=w509:u8)
                n186 = Index Array(array=w515, index=2 ("索引")) -> (element=w507:u8)
                n187 = Index Array(array=w515, index=3 ("索引")) -> (element=w505:u8)
                n188 = Index Array(array=w515, index=0 ("索引")) -> (element=w510:u8)
                n189 = Number To Boolean Array(number=w509) -> (Boolean array=w508:bool[])
                n190 = Number To Boolean Array(number=w507) -> (Boolean array=w506:bool[])
                n191 = Number To Boolean Array(number=w505) -> (Boolean array=w504:bool[])
                n192 = Number To Boolean Array(number=w510) -> (Boolean array=w522:bool[])
                n193 = Index Array(array=w522, index=5 ("索引")) -> (element=→"I0.5":bool)
                n194 = Index Array(array=w522, index=6 ("索引")) -> (element=→"I0.6":bool)
                n195 = Index Array(array=w522, index=7 ("索引")) -> (element=→"I0.7":bool)
                n196 = Index Array(array=w522, index=2 ("索引")) -> (element=→"I0.2":bool)
                n197 = Index Array(array=w522, index=3 ("索引")) -> (element=→"I0.3":bool)
                n198 = Index Array(array=w522, index=4 ("索引")) -> (element=→"I0.4":bool)
                n199 = Index Array(array=w522, index=0 ("索引")) -> (element=→"I0.0":bool)
                n200 = Index Array(array=w522, index=1 ("索引")) -> (element=→"I0.1":bool)
              }
              frame #1 {
                n201 = Index Array(array=w533, index=1 ("索引")) -> (element=→"I1.1":bool)
                n202 = Index Array(array=w533, index=2 ("索引")) -> (element=→"I1.2":bool)
                n203 = Index Array(array=w533, index=7 ("索引")) -> (element=→"I1.7":bool)
                n204 = Index Array(array=w533, index=4 ("索引")) -> (element=→"I1.4":bool)
                n205 = Index Array(array=w533, index=6 ("索引")) -> (element=→"I1.6":bool)
                n206 = Index Array(array=w533, index=3 ("索引")) -> (element=→"I1.3":bool)
                n207 = Index Array(array=w533, index=0 ("索引")) -> (element=→"I1.0":bool)
                n208 = Index Array(array=w533, index=5 ("索引")) -> (element=→"I1.5":bool)
              }
              frame #2 {
                n209 = Index Array(array=w550, index=5 ("索引")) -> (element=→"I2.5":bool)
                n210 = Index Array(array=w550, index=6 ("索引")) -> (element=→"I2.6":bool)
                n211 = Index Array(array=w550, index=7 ("索引")) -> (element=→"I2.7":bool)
                n212 = Index Array(array=w550, index=2 ("索引")) -> (element=→"I2.2":bool)
                n213 = Index Array(array=w550, index=3 ("索引")) -> (element=→"I2.3":bool)
                n214 = Index Array(array=w550, index=4 ("索引")) -> (element=→"I2.4":bool)
                n215 = Index Array(array=w550, index=0 ("索引")) -> (element=→"I2.0":bool)
                n216 = Index Array(array=w550, index=1 ("索引")) -> (element=→"I2.1":bool)
              }
              frame #3 {
                n217 = Index Array(array=w567, index=1 ("索引")) -> (element=→"I3.1":bool)
                n218 = Index Array(array=w567, index=5 ("索引")) -> (element=→"I3.5":bool)
                n219 = Index Array(array=w567, index=6 ("索引")) -> (element=→"I3.6":bool)
                n220 = Index Array(array=w567, index=7 ("索引")) -> (element=→"I3.7":bool)
                n221 = Index Array(array=w567, index=2 ("索引")) -> (element=→"I3.2":bool)
                n222 = Index Array(array=w567, index=3 ("索引")) -> (element=→"I3.3":bool)
                n223 = Index Array(array=w567, index=4 ("索引")) -> (element=→"I3.4":bool)
                n224 = Index Array(array=w567, index=0 ("索引")) -> (element=→"I3.0":bool)
              }
            }
          }
          frame "枚举RQ" {
            n225 = stacked-sequence {
              seq-local: [w589 _ _ _] -> [_ w614 _ _]
              seq-local: [w587 _ _ _] -> [_ _ w631 _]
              seq-local: [w585 _ _ _] -> [_ _ _ w648]
              tunnel: w584 -> [w596 _ _ _]
              frame #0 {
                n226 = Index Array(array=w596, index=1 ("索引")) -> (element=w590:u8)
                n227 = Index Array(array=w596, index=2 ("索引")) -> (element=w588:u8)
                n228 = Index Array(array=w596, index=3 ("索引")) -> (element=w586:u8)
                n229 = Index Array(array=w596, index=0 ("索引")) -> (element=w591:u8)
                n230 = Number To Boolean Array(number=w590) -> (Boolean array=w589:bool[])
                n231 = Number To Boolean Array(number=w588) -> (Boolean array=w587:bool[])
                n232 = Number To Boolean Array(number=w586) -> (Boolean array=w585:bool[])
                n233 = Number To Boolean Array(number=w591) -> (Boolean array=w603:bool[])
                n234 = Index Array(array=w603, index=5 ("索引")) -> (element=→"Q0.5":bool)
                n235 = Index Array(array=w603, index=6 ("索引")) -> (element=→"Q0.6":bool)
                n236 = Index Array(array=w603, index=7 ("索引")) -> (element=→"Q0.7":bool)
                n237 = Index Array(array=w603, index=2 ("索引")) -> (element=→"Q0.2":bool)
                n238 = Index Array(array=w603, index=3 ("索引")) -> (element=→"Q0.3":bool)
                n239 = Index Array(array=w603, index=4 ("索引")) -> (element=→"Q0.4":bool)
                n240 = Index Array(array=w603, index=0 ("索引")) -> (element=→"Q0.0":bool)
                n241 = Index Array(array=w603, index=1 ("索引")) -> (element=→"Q0.1":bool)
              }
              frame #1 {
                n242 = Index Array(array=w614, index=1 ("索引")) -> (element=→"Q1.1":bool)
                n243 = Index Array(array=w614, index=2 ("索引")) -> (element=→"Q1.2":bool)
                n244 = Index Array(array=w614, index=7 ("索引")) -> (element=→"Q1.7":bool)
                n245 = Index Array(array=w614, index=4 ("索引")) -> (element=→"Q1.4":bool)
                n246 = Index Array(array=w614, index=6 ("索引")) -> (element=→"Q1.6":bool)
                n247 = Index Array(array=w614, index=3 ("索引")) -> (element=→"Q1.3":bool)
                n248 = Index Array(array=w614, index=0 ("索引")) -> (element=→"Q1.0":bool)
                n249 = Index Array(array=w614, index=5 ("索引")) -> (element=→"Q1.5":bool)
              }
              frame #2 {
                n250 = Index Array(array=w631, index=5 ("索引")) -> (element=→"Q2.5":bool)
                n251 = Index Array(array=w631, index=6 ("索引")) -> (element=→"Q2.6":bool)
                n252 = Index Array(array=w631, index=7 ("索引")) -> (element=→"Q2.7":bool)
                n253 = Index Array(array=w631, index=2 ("索引")) -> (element=→"Q2.2":bool)
                n254 = Index Array(array=w631, index=3 ("索引")) -> (element=→"Q2.3":bool)
                n255 = Index Array(array=w631, index=4 ("索引")) -> (element=→"Q2.4":bool)
                n256 = Index Array(array=w631, index=0 ("索引")) -> (element=→"Q2.0":bool)
                n257 = Index Array(array=w631, index=1 ("索引")) -> (element=→"Q2.1":bool)
              }
              frame #3 {
                n258 = Index Array(array=w648, index=1 ("索引")) -> (element=→"Q3.1":bool)
                n259 = Index Array(array=w648, index=5 ("索引")) -> (element=→"Q3.5":bool)
                n260 = Index Array(array=w648, index=6 ("索引")) -> (element=→"Q3.6":bool)
                n261 = Index Array(array=w648, index=7 ("索引")) -> (element=→"Q3.7":bool)
                n262 = Index Array(array=w648, index=2 ("索引")) -> (element=→"Q3.2":bool)
                n263 = Index Array(array=w648, index=3 ("索引")) -> (element=→"Q3.3":bool)
                n264 = Index Array(array=w648, index=4 ("索引")) -> (element=→"Q3.4":bool)
                n265 = Index Array(array=w648, index=0 ("索引")) -> (element=→"Q3.0":bool)
              }
            }
          }
          frame "枚举RM" {
            n266 = stacked-sequence {
              seq-local: [w671 _ _ _] -> [_ w695 _ _]
              seq-local: [w669 _ _ _] -> [_ _ w712 _]
              seq-local: [w667 _ _ _] -> [_ _ _ w729]
              tunnel: w665 -> [w666 _ _ _]
              frame #0 {
                n267 = Index Array(array=w666, index=1 ("索引")) -> (element=w672:u8)
                n268 = Index Array(array=w666, index=2 ("索引")) -> (element=w670:u8)
                n269 = Index Array(array=w666, index=3 ("索引")) -> (element=w668:u8)
                n270 = Index Array(array=w666, index=0 ("索引")) -> (element=w673:u8)
                n271 = Number To Boolean Array(number=w672) -> (Boolean array=w671:bool[])
                n272 = Number To Boolean Array(number=w670) -> (Boolean array=w669:bool[])
                n273 = Number To Boolean Array(number=w668) -> (Boolean array=w667:bool[])
                n274 = Number To Boolean Array(number=w673) -> (Boolean array=w684:bool[])
                n275 = Index Array(array=w684, index=6 ("索引")) -> (element=→"M0.6":bool)
                n276 = Index Array(array=w684, index=7 ("索引")) -> (element=→"M0.7":bool)
                n277 = Index Array(array=w684, index=2 ("索引")) -> (element=→"M0.2":bool)
                n278 = Index Array(array=w684, index=3 ("索引")) -> (element=→"M0.3":bool)
                n279 = Index Array(array=w684, index=4 ("索引")) -> (element=→"M0.4":bool)
                n280 = Index Array(array=w684, index=0 ("索引")) -> (element=→"M0.0":bool)
                n281 = Index Array(array=w684, index=1 ("索引")) -> (element=→"M0.1":bool)
                n282 = Index Array(array=w684, index=5 ("索引")) -> (element=→"M0.5":bool)
              }
              frame #1 {
                n283 = Index Array(array=w695, index=1 ("索引")) -> (element=→"M1.1":bool)
                n284 = Index Array(array=w695, index=2 ("索引")) -> (element=→"M1.2":bool)
                n285 = Index Array(array=w695, index=7 ("索引")) -> (element=→"M1.7":bool)
                n286 = Index Array(array=w695, index=4 ("索引")) -> (element=→"M1.4":bool)
                n287 = Index Array(array=w695, index=6 ("索引")) -> (element=→"M1.6":bool)
                n288 = Index Array(array=w695, index=3 ("索引")) -> (element=→"M1.3":bool)
                n289 = Index Array(array=w695, index=0 ("索引")) -> (element=→"M1.0":bool)
                n290 = Index Array(array=w695, index=5 ("索引")) -> (element=→"M1.5":bool)
              }
              frame #2 {
                n291 = Index Array(array=w712, index=5 ("索引")) -> (element=→"M2.5":bool)
                n292 = Index Array(array=w712, index=6 ("索引")) -> (element=→"M2.6":bool)
                n293 = Index Array(array=w712, index=7 ("索引")) -> (element=→"M2.7":bool)
                n294 = Index Array(array=w712, index=2 ("索引")) -> (element=→"M2.2":bool)
                n295 = Index Array(array=w712, index=3 ("索引")) -> (element=→"M2.3":bool)
                n296 = Index Array(array=w712, index=4 ("索引")) -> (element=→"M2.4":bool)
                n297 = Index Array(array=w712, index=0 ("索引")) -> (element=→"M2.0":bool)
                n298 = Index Array(array=w712, index=1 ("索引")) -> (element=→"M2.1":bool)
              }
              frame #3 {
                n299 = Index Array(array=w729, index=1 ("索引")) -> (element=→"Q3.1":bool)
                n300 = Index Array(array=w729, index=5 ("索引")) -> (element=→"Q3.5":bool)
                n301 = Index Array(array=w729, index=6 ("索引")) -> (element=→"Q3.6":bool)
                n302 = Index Array(array=w729, index=7 ("索引")) -> (element=→"Q3.7":bool)
                n303 = Index Array(array=w729, index=2 ("索引")) -> (element=→"Q3.2":bool)
                n304 = Index Array(array=w729, index=3 ("索引")) -> (element=→"Q3.3":bool)
                n305 = Index Array(array=w729, index=4 ("索引")) -> (element=→"Q3.4":bool)
                n306 = Index Array(array=w729, index=0 ("索引")) -> (element=→"Q3.0":bool)
              }
            }
          }
          frame "枚举RVW" {
            n307 = String Subset(string=w747, offset (0)=25 ("偏移量(0)"), length (rest)=40 ("长度（剩余）")) -> (substring=w746:string)
            n308 = stacked-sequence {
              tunnel: w746 -> [w750 w805]
              frame #0 {
                n309 = String Subset(string=w750, offset (0)=6 ("偏移量(0)"), length (rest)=8 ("长度（剩余）")) -> (substring=w782:string)
                n310 = String Subset(string=w750, offset (0)=0 ("偏移量(0)"), length (rest)=2 ("长度（剩余）")) -> (substring=w791:string)
                n311 = String Subset(string=w750, offset (0)=2 ("偏移量(0)"), length (rest)=4 ("长度（剩余）")) -> (substring=w790:string)
                n312 = String Subset(string=w750, offset (0)=4 ("偏移量(0)"), length (rest)=6 ("长度（剩余）")) -> (substring=w783:string)
                n313 = String Subset(string=w750, offset (0)=8 ("偏移量(0)"), length (rest)=10 ("长度（剩余）")) -> (substring=w775:string)
                n314 = String Subset(string=w750, offset (0)=16 ("偏移量(0)"), length (rest)=18 ("长度（剩余）")) -> (substring=w753:string)
                n315 = String Subset(string=w750, offset (0)=10 ("偏移量(0)"), length (rest)=12 ("长度（剩余）")) -> (substring=w774:string)
                n316 = String Subset(string=w750, offset (0)=12 ("偏移量(0)"), length (rest)=14 ("长度（剩余）")) -> (substring=w767:string)
                n317 = String Subset(string=w750, offset (0)=14 ("偏移量(0)"), length (rest)=16 ("长度（剩余）")) -> (substring=w766:string)
                n318 = Type Cast(type=u16 0, x=w782) -> (*(type *) &x=→"RVW6":u16)
                n319 = Type Cast(type=u16 0, x=w791) -> (*(type *) &x=→"RVW0":u16)
                n320 = Type Cast(type=u16 0, x=w790) -> (*(type *) &x=→"RVW2":u16)
                n321 = Type Cast(type=u16 0, x=w783) -> (*(type *) &x=→"RVW4":u16)
                n322 = Type Cast(type=u16 0, x=w775) -> (*(type *) &x=→"RVW8":u16)
                n323 = Type Cast(type=u16 0, x=w753) -> (*(type *) &x=→"RVW16":u16)
                n324 = Type Cast(type=u16 0, x=w774) -> (*(type *) &x=→"RVW10":u16)
                n325 = Type Cast(type=u16 0, x=w767) -> (*(type *) &x=→"RVW12":u16)
                n326 = Type Cast(type=u16 0, x=w766) -> (*(type *) &x=→"RVW14":u16)
              }
              frame #1 {
                n327 = String Subset(string=w805, offset (0)=18 ("偏移量(0)"), length (rest)=20 ("长度（剩余）")) -> (substring=w838:string)
                n328 = String Subset(string=w805, offset (0)=20 ("偏移量(0)"), length (rest)=22 ("长度（剩余）")) -> (substring=w837:string)
                n329 = String Subset(string=w805, offset (0)=22 ("偏移量(0)"), length (rest)=24 ("长度（剩余）")) -> (substring=w830:string)
                n330 = String Subset(string=w805, offset (0)=24 ("偏移量(0)"), length (rest)=26 ("长度（剩余）")) -> (substring=w829:string)
                n331 = String Subset(string=w805, offset (0)=26 ("偏移量(0)"), length (rest)=28 ("长度（剩余）")) -> (substring=w822:string)
                n332 = String Subset(string=w805, offset (0)=28 ("偏移量(0)"), length (rest)=30 ("长度（剩余）")) -> (substring=w821:string)
                n333 = String Subset(string=w805, offset (0)=30 ("偏移量(0)"), length (rest)=32 ("长度（剩余）")) -> (substring=w814:string)
                n334 = String Subset(string=w805, offset (0)=32 ("偏移量(0)"), length (rest)=34 ("长度（剩余）")) -> (substring=w813:string)
                n335 = String Subset(string=w805, offset (0)=34 ("偏移量(0)"), length (rest)=36 ("长度（剩余）")) -> (substring=w806:string)
                n336 = Type Cast(type=u16 0, x=w838) -> (*(type *) &x=→"RVW18":u16)
                n337 = Type Cast(type=u16 0, x=w837) -> (*(type *) &x=→"RVW20":u16)
                n338 = Type Cast(type=u16 0, x=w830) -> (*(type *) &x=→"RVW22":u16)
                n339 = Type Cast(type=u16 0, x=w829) -> (*(type *) &x=→"RVW24":u16)
                n340 = Type Cast(type=u16 0, x=w822) -> (*(type *) &x=→"RVW26":u16)
                n341 = Type Cast(type=u16 0, x=w821) -> (*(type *) &x=→"RVW28":u16)
                n342 = Type Cast(type=u16 0, x=w814) -> (*(type *) &x=→"RVW30":u16)
                n343 = Type Cast(type=u16 0, x=w813) -> (*(type *) &x=→"RVW32":u16)
                n344 = Type Cast(type=u16 0, x=w806) -> (*(type *) &x=→"RVW34":u16)
              }
            }
          }
          frame "WID0" {
          }
          frame "WQD0" {
          }
          frame "WMD0" {
          }
          frame "WV" {
          }
          frame "STOP" {
          }
          frame "RUN" {
          }
          frame "捂手" {
          }
        }
      }
    }
  }
  n345 = VISA Flush I/O Buffer(VISA resource name=w5, error in (no error)=w4) -> (VISA resource name out=w3:refnum<visa-resource-name>, error out=w2:errorcluster)  [unwired: 1 in]
  n346 = VISA Close(VISA resource name=w3, error in (no error)=w2) -> ()  [unwired: 1 out]
